vi "移动窗口.vi"() -> ()   [LabVIEW 2018]
uses:
  Windows/System32/user32.dll
panel:
  in  "停止":bool
  out "透明标题栏":string
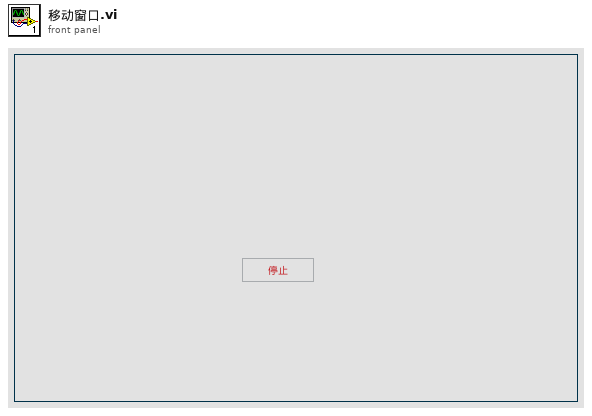
[diagram p1: front panel]
types:
  T1 = enum32{"Invalid", "Standard", "Closed", "Hidden", "Minimized", "Maximized"}
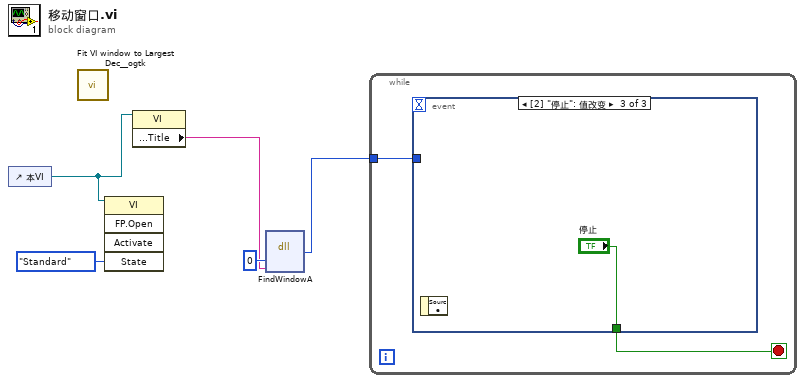
[diagram p0: block diagram]
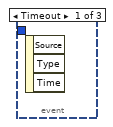
[diagram p2: hidden frame]
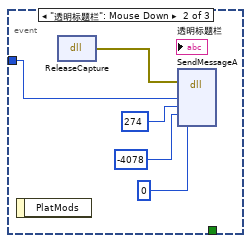
[diagram p3: hidden frame]
diagram:
  n1 = control-ref of="本VI"() -> (w4:refnum<vi>)
  n2 = call <userlib>:"Fit VI window to Largest Dec__ogtk.vi"() -> ()  [unwired: 6 in, 2 out]
  n3 = invoke class="VI" method="FP.Open"(reference=w4, "State"=T1."Standard" ("状态")) -> ()  [unwired: 3 in, 5 out]
  n4 = property class="VI"(reference=w4) -> ("Front Panel.Title"=w2:string)  [unwired: 1 in, 2 out]
  n5 = dll-call lib="C:/Windows/System32/user32.dll" fn="FindWindowA"("IpClassName"=0, "Ipwindowname"=w2) -> ("HWND"=w1:u32)  [unwired: 5 in, 2 out]
  n6 = while {
    tunnel: w1 -> [w7]
    stop <- w6 stop-if-true
    n7 = event shown="[2] \"停止\": 值改变" {
      selector: _ -> [_ _ _]
      dyn-events: _ -> [_ _ _]
      timeout: _ -> [_ _ _]
      tunnel: w7 -> [_ w11 _]
      tunnel: [_ _ "停止"] -> w6
      event Timeout {
        n8 = event-data() -> ()  [unwired: 1 in, 3 out]
      }
      event "透明标题栏": Mouse Down {
        n9 = event-data() -> ()  [unwired: 1 in, 1 out]
        n10 = dll-call lib="C:/Windows/System32/user32.dll" fn="ReleaseCapture"() -> (error out=w12:errorcluster)  [unwired: 4 in, 1 out]
        n11 = dll-call lib="C:/Windows/System32/user32.dll" fn="SendMessageA"(error in=w12, "参数1"=w11, "参数2"=i16 274, "参数3"=i16 -4078 ("参数2"), "参数4"=i16 0 ("参数2")) -> ()  [unwired: 7 in, 2 out]
      }
      event "停止": Value Change {
        n12 = event-data() -> ()  [unwired: 1 in, 1 out]
      }
    }
  }
